vi "Impulse_Correlation.vi"(0 "Head Velocity":dbl[][](array[numeric])=array6400x4[25600 elements] format="%.2f", 2 "Trigger":T1(ring)=enum."Falling Edge", 5 "Cross-Correlation":bool, 7 "Impulse surround":T2={"Pre Impulse (ms)"=150, "Post Impulse (ms) "=150, "Pitch/Roll T for RALP/LARP"=15.0} {"Pitch/Roll T for RALP/LARP" format="%.2f"}, 9 "First Pass Criterea":T5={"Minimum Threshold"=100.0, "Width (ms)"=50, "Maximum Threshold"=100.0} {"Maximum Threshold" format="%.2f"; "Minimum Threshold" format="%.2f"}, 11 "Sample Rate":dbl format="%.2f", 12 "Other Trigger":bool) -> (4 "Impulse Array":T6(array[cluster]) {"Amplitude offset" format="%.2f"})   [LabVIEW 2013, in "impulse functions.lvlib"]
uses:
  impulse functions.lvlib
  <vilib>/Analysis/2dsp.llb/1D Cross Correlation (DBL).vi
  <vilib>/Analysis/NI_AALPro.lvlib
  <vilib>/Analysis/NI_AALBase.lvlib
  <vilib>/Analysis/3filter.llb/Savitzky-Golay Filter (DBL).vi
panel:
  out "extracted head impulse 3":dbl[][](graph)
  out "extracted head impulse 2":dbl[](graph)
  out "extracted head impulse":dbl[][](graph)
  in  "Peaks/Valleys":enum16{"Peaks", "Valleys"}(ring)
  in  "Impulse":T3 {"Amplitude offset" format="%.2f"}
  in  "Impulse Analysis Params":T4={"unfiltered vel?"=FALSE, "remove offset? (T)"=FALSE, "analysis method"=enum."polynomial fit", "pre-impulse position"=50, "post-impulse position"=50, "HIT axis"=enum."Pitch", "pre-impulse pts"=50, "post-impulse pts"=50, "polynomial order"=15, "algorithm"=enum."Givens"}
  # "Copyright Americo A. Migliaccio (c) 2002 All Rights Reserved by Author"
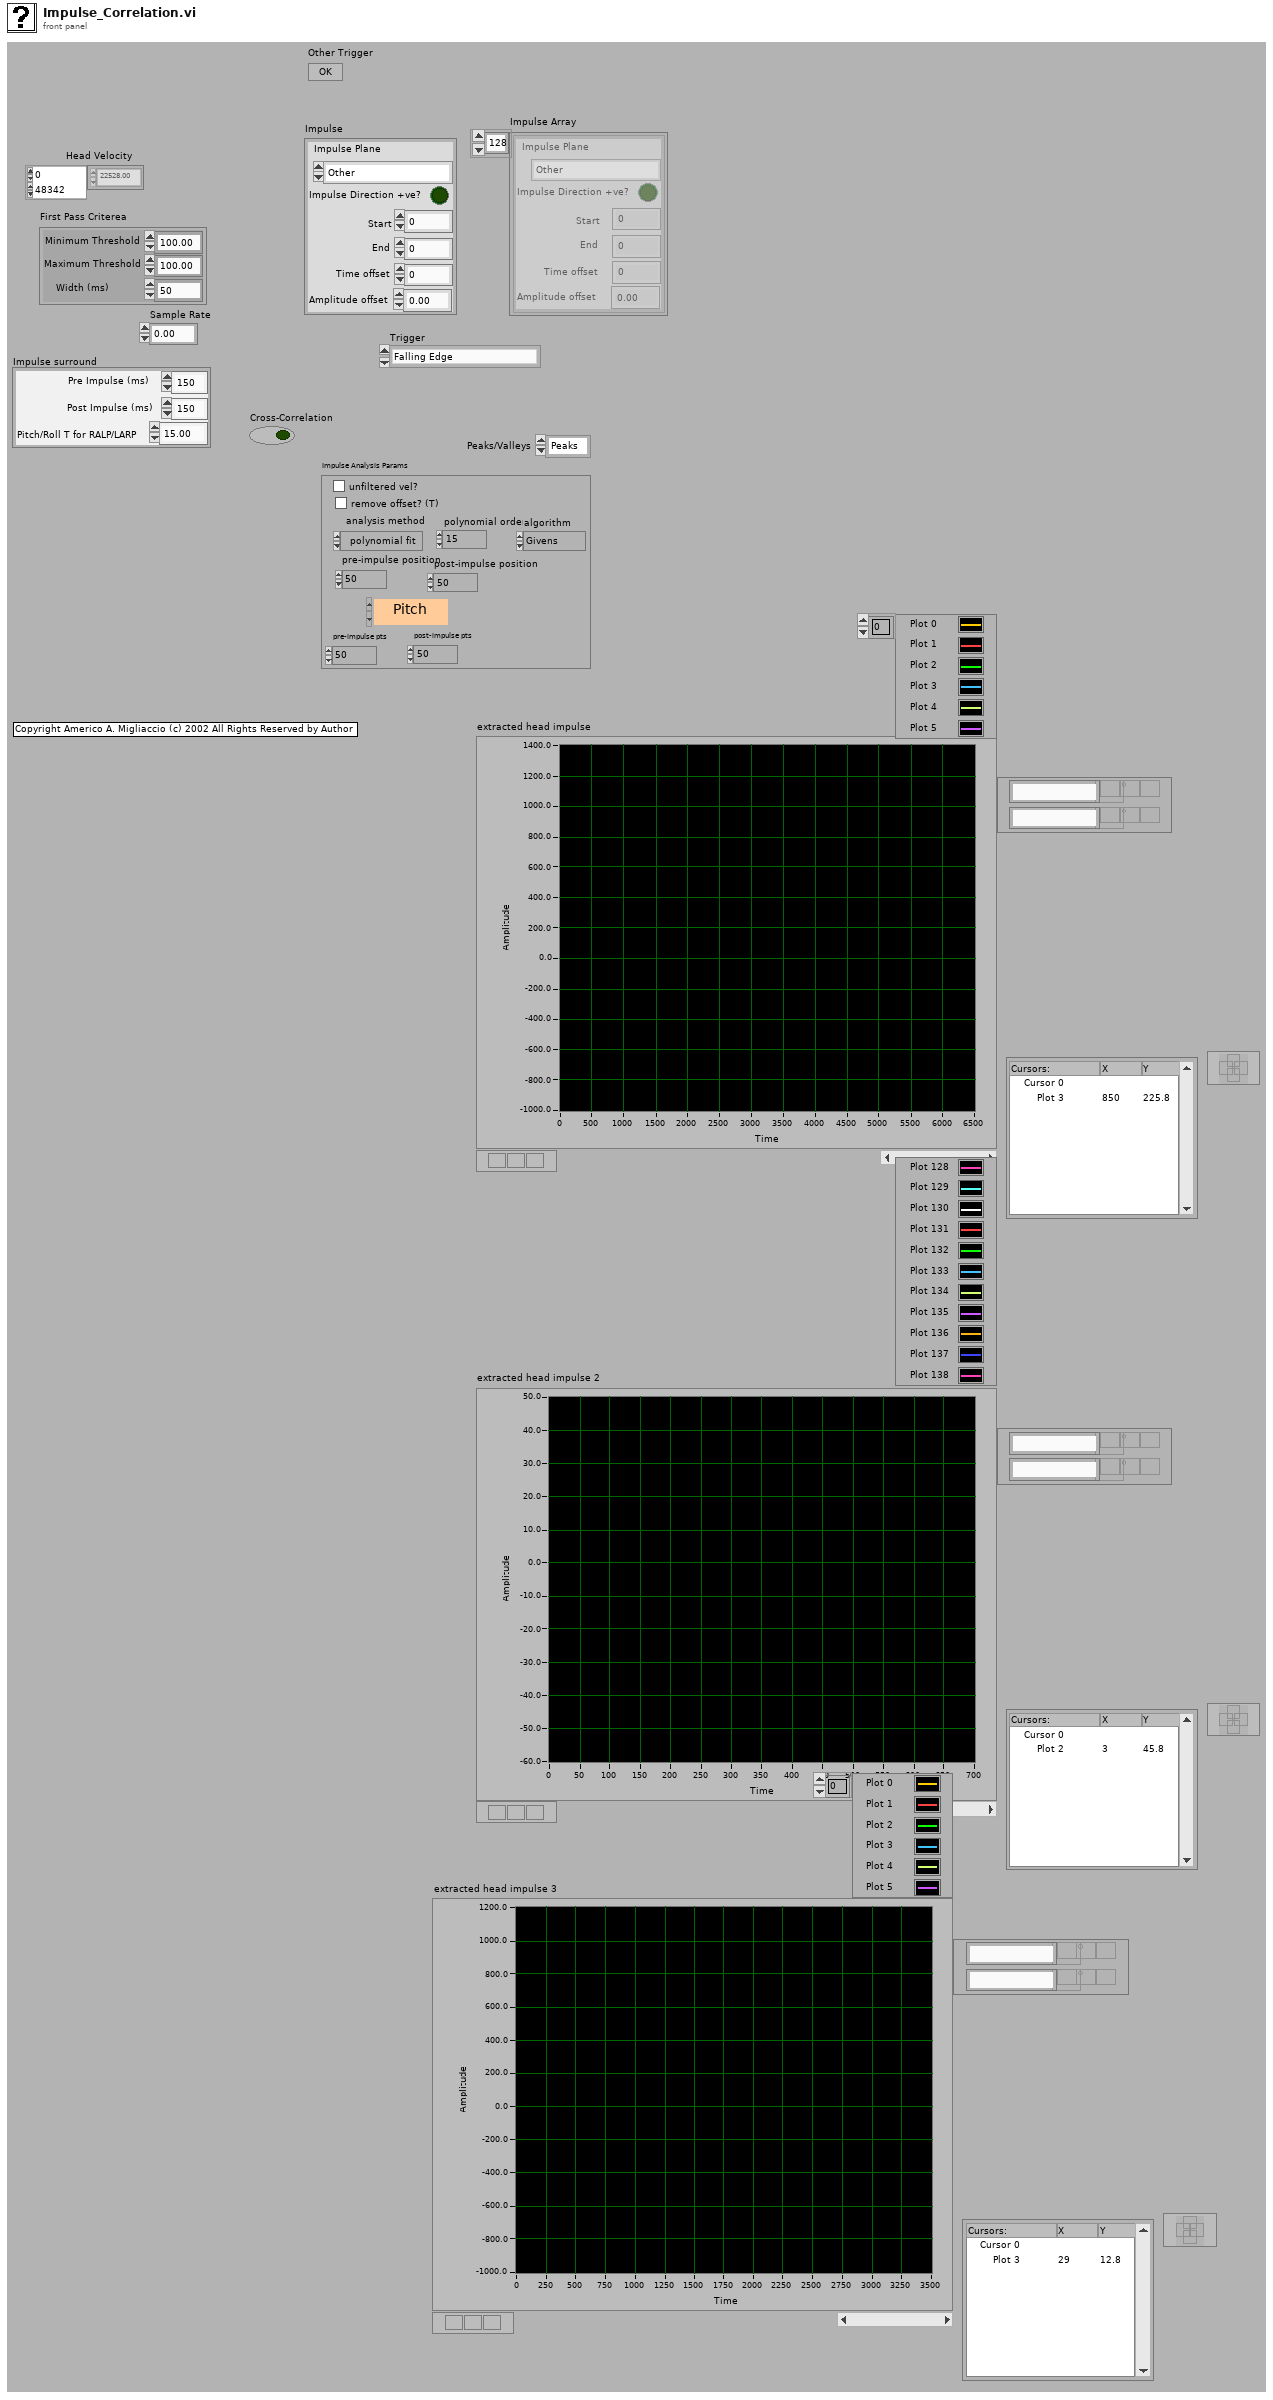
[diagram p1: front panel]
types:
  T1 = enum16{"Peak Detektion", "Rising Edge", "Falling Edge", "Rising Edge (multiple)", "Falling Edge (multiple)"}
  T2 = cluster{"Pre Impulse (ms)":i32, "Post Impulse (ms) ":i32, "Pitch/Roll T for RALP/LARP":dbl}
  T3 = cluster{"Start":i32, "End":i32, "Impulse Plane":enum16{"Other", "Yaw", "Pitch", "Roll", "LARP", "RALP"}, "Impulse Direction +ve?":bool, "Time offset":i32, "Amplitude offset":dbl}
  T4 = cluster{"unfiltered vel?":bool, "remove offset? (T)":bool, "analysis method":enum16{"original", "polynomial fit"}, "pre-impulse position":i32, "post-impulse position":i32, "HIT axis":enum16{"Yaw", "Pitch", "Roll"}, "pre-impulse pts":i32, "post-impulse pts":i32, "polynomial order":i32, "algorithm":enum32{"SVD", "Givens", "Givens2", "Householder", "LU Decomposition", "Cholesky"}}
  T5 = cluster{"Minimum Threshold":dbl, "Width (ms)":i32, "Maximum Threshold":dbl}
  T6 = cluster{"Start":i32, "End":i32, "Impulse Plane":enum16{"Other", "Yaw", "Pitch", "Roll", "LARP", "RALP"}, "Impulse Direction +ve?":bool, "Time offset":i32, "Amplitude offset":dbl}[]
  T7 = cluster{"baseline intercept":dbl, "impulse peak X":dbl, "len":i32, "+ve ?":bool, "peak velocity":dbl}
  T8 = enum16{"Other", "Yaw", "Pitch", "Roll", "LARP", "RALP"}
  T9 = cluster{"Impulse Plane":enum16{"Other", "Yaw", "Pitch", "Roll", "LARP", "RALP"}, "Impulse Direction +ve?":bool}
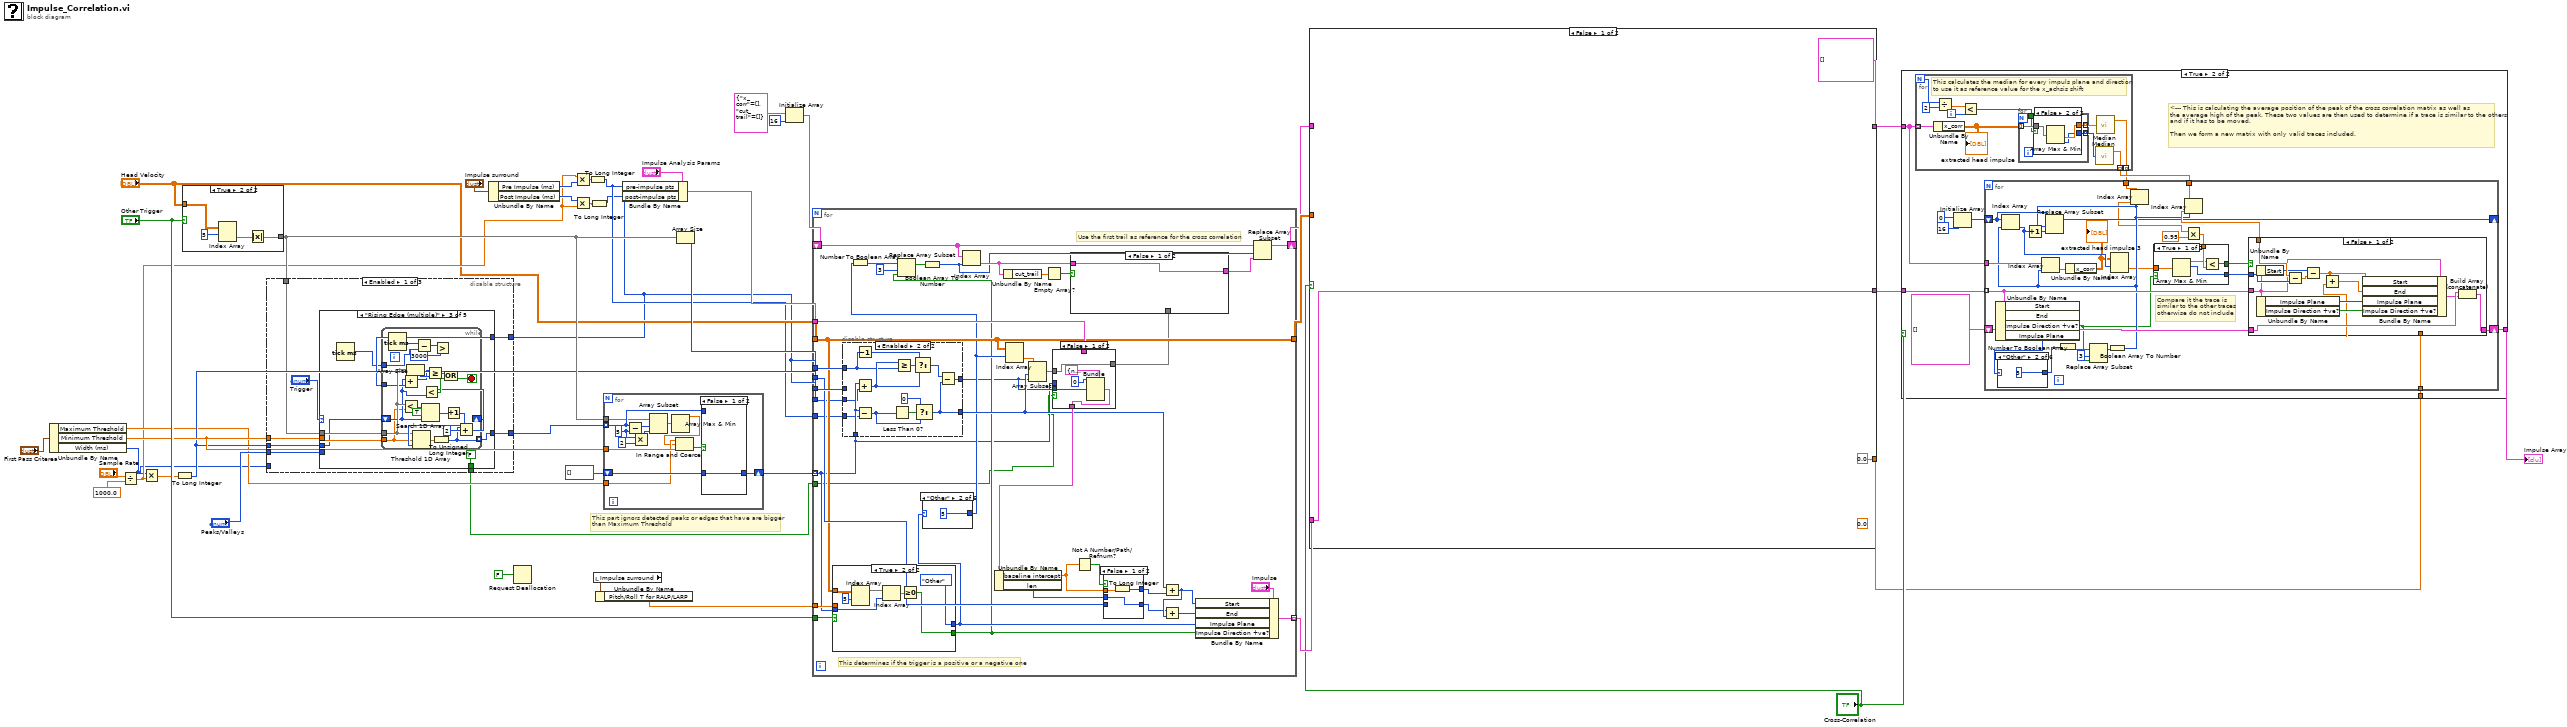
[diagram p0: block diagram]
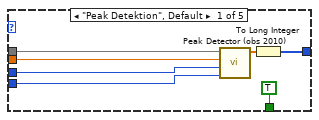
[diagram p2: hidden frame]
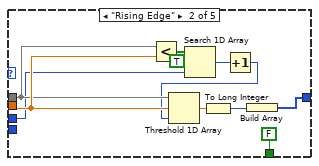
[diagram p3: hidden frame]
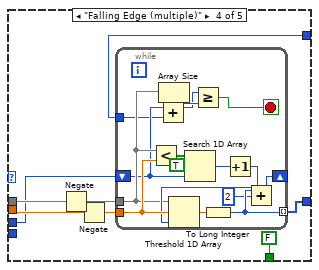
[diagram p4: hidden frame]
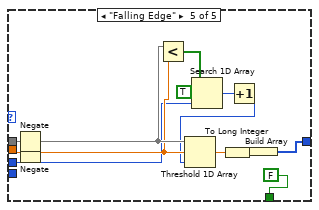
[diagram p5: hidden frame]
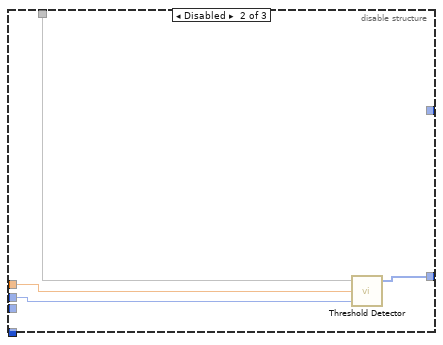
[diagram p6: hidden frame]
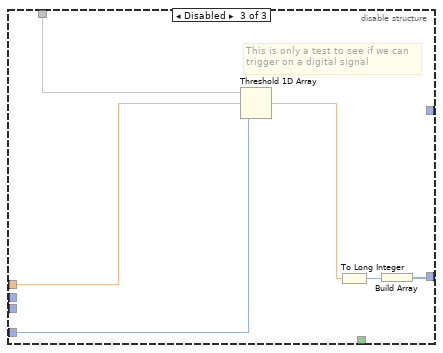
[diagram p7: hidden frame]
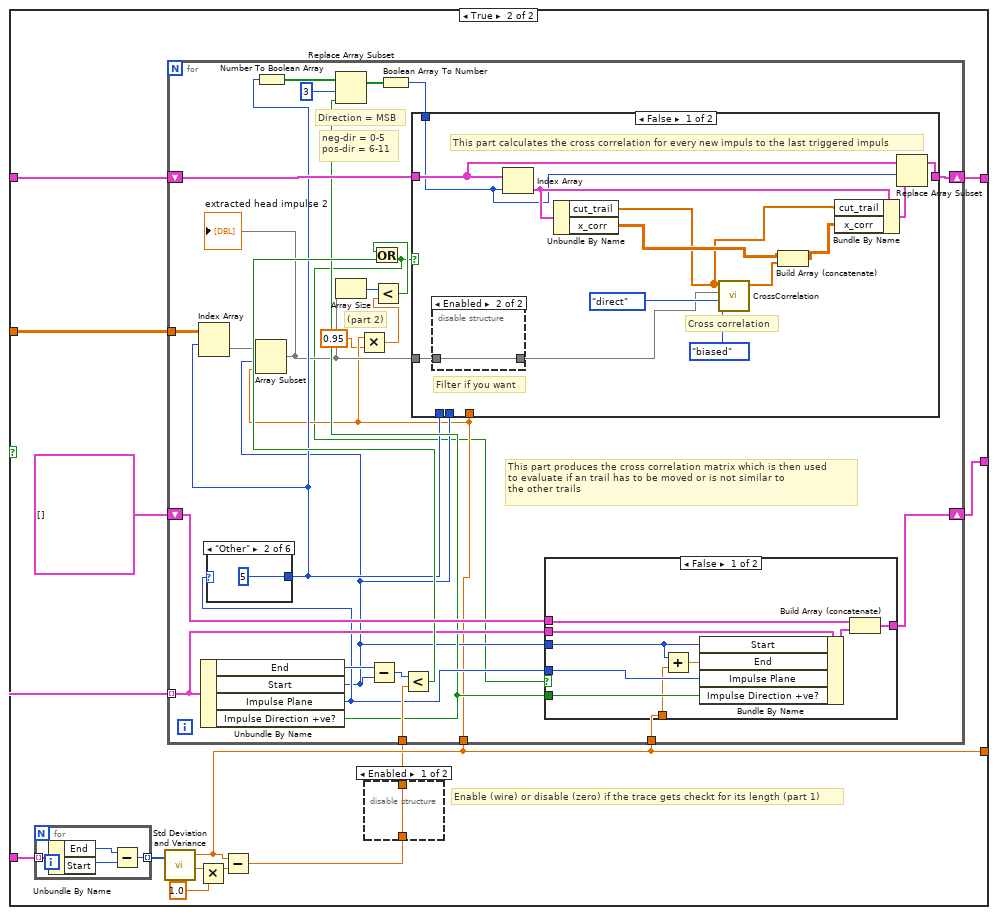
[diagram p8: hidden frame]
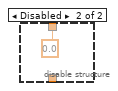
[diagram p9: hidden frame]
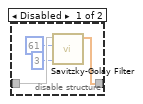
[diagram p10: hidden frame]
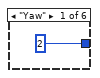
[diagram p12: hidden frame]
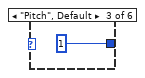
[diagram p13: hidden frame]
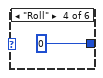
[diagram p14: hidden frame]
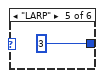
[diagram p15: hidden frame]
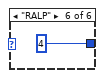
[diagram p16: hidden frame]
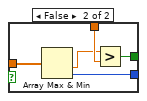
[diagram p19: hidden frame]
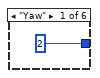
[diagram p20: hidden frame]
diagram:
  # "This part ignors detected peaks or edges that have are bigger \nthan Maximum Threshold"
  n1 = Unbundle By Name("First Pass Criterea") -> ("Maximum Threshold"=w24:dbl, "Minimum Threshold"=w29:dbl, "Width (ms)"=w5:i32)
  n2 = Divide(x="Sample Rate", y=1000.0 ("x")) -> (x/y=w19:dbl)
  n3 = Multiply(x=w5, y=w19) -> (x*y=w18:dbl)
  n4 = To Long Integer(number=w18) -> (32bit integer=w27:i32)
  n5 = case shown="True" "Other Trigger" {
    tunnel: [w46 w47] -> w36
    tunnel: "Head Velocity" -> [w42 w49]
    frame False {
      n6 = Array Subset(array=w42, index (row)=0 ("Array Index"), length (row)=3 ("Array Length")) -> (w43:dbl[][])  [unwired: 2 in]
      n7 = call "norm 3D array.vi"("Vector"=w43) -> ("|x|"=w46:dbl[])  [unwired: 1 in, 1 out]
    }
    frame True {
      n8 = Index Array(array=w49, index (row)=5 ("Array Index")) -> (element=w48:dbl[])  [unwired: 1 in]
      n9 = Absolute Value(x=w48) -> (abs(x)=w47:dbl[])
    }
  }
  n10 = Unbundle By Name("Impulse surround") -> ("Pre Impulse (ms)"=w21:i32, "Post Impulse (ms)"=w20:i32)
  n11 = Request Deallocation(FALSE ("flag")) -> ()
  n12 = Multiply(x=w19, y=w21) -> (x*y=w22:dbl)
  n13 = Multiply(x=w20, y=w19) -> (x*y=w23:dbl)
  n14 = To Long Integer(number=w22) -> (32bit integer=w3:i32)
  n15 = To Long Integer(number=w23) -> (32bit integer=w1:i32)
  n16 = disable-structure shown="Enabled" {
    disable-tunnel: [w58 w141 w148] -> w41
    disable-tunnel: w36 -> [w57 w144 w150]
    disable-tunnel: w29 -> [w56 w143 w149]
    disable-tunnel: "Peaks/Valleys" -> [w55 _ _]
    disable-tunnel: w27 -> [w54 w142 _]
    disable-tunnel: w5 -> [_ _ w145]
    disable-tunnel: [w52 _ _] -> w2
    disable-tunnel: w1 -> [w51 _ _]
    frame Enabled {
      n17 = case shown="\"Rising Edge (multiple)\"" "Trigger" {
        tunnel: [w64 w74 w83 w112 w137] -> w58
        tunnel: w57 -> [w63 w69 w80 w109 w133]
        tunnel: w56 -> [w62 w72 w81 w110 w138]
        tunnel: w55 -> [w61 _ _ _ _]
        tunnel: w54 -> [w60 w68 w79 w108 w130]
        tunnel: [TRUE FALSE FALSE FALSE FALSE] -> w52
        tunnel: w51 -> [_ _ w78 w105 _]
        frame "Peak Detektion", Default {
          n18 = call <vilib>:"Peak Detector (obs 2010).vi"("peaks/valleys"=w61, "width"=w60, "threshold"=w62, "X"=w63) -> ("Locations"=w65:dbl[])  [unwired: 3 in, 4 out]
          n19 = To Long Integer(number=w65) -> (32bit integer=w64:i32[])
        }
        frame "Rising Edge" {
          n20 = Less?(x=w69, y=w72) -> (x < y?=w71:bool[])
          n21 = Search 1D Array(1D array=w71, element=TRUE, start index (0)=w68) -> (index of element=w67:i32)
          n22 = Increment(x=w67) -> (x+1=w66:i32)
          n23 = Threshold 1D Array(1:w66, 2:w72, 3:w69) -> (0:w76:dbl)
          n24 = To Long Integer(number=w76) -> (32bit integer=w75:i32)
          n25 = Build Array(w75) -> (w74:i32[])
        }
        frame "Rising Edge (multiple)" {
          n26 = Tick Count (ms)() -> (millisecond timer value=w77:u32)
          n27 = while {
            tunnel: [w85] -> w83 mode=indexing
            tunnel: w81 -> [w86]
            tunnel: w80 -> [w99]
            shift-right: [w84] -> _
            shift-left: w79 -> [w94]
            tunnel: w78 -> [w95]
            tunnel: w77 -> [w91]
            stop <- w87 stop-if-true
            n28 = Tick Count (ms)() -> (millisecond timer value=w90:u32)
            n29 = Add(x=w94, y=w95) -> (x+y=w96:u32)
            n30 = Less?(x=w99, y=w86) -> (x < y?=w103:bool[])
            n31 = Array Size(array=w99) -> (size(s)=w98:i32)
            n32 = Subtract(x=w90, y=w91) -> (x-y=w89:u32)
            n33 = Search 1D Array(1D array=w103, element=TRUE, start index (0)=w94) -> (index of element=w101:i32)
            n34 = Greater Or Equal?(x=w96, y=w98) -> (x >= y?=w93:bool)
            n35 = Greater?(x=w89, y=u32 3000) -> ()  [unwired: 1 out]
            n36 = Increment(x=w101) -> (x+1=w100:i32)
            n37 = Threshold 1D Array(1:w100, 2:w86, 3:w99) -> (0:w104:dbl)
            n38 = To Unsigned Long Integer(number=w104) -> (unsigned 32bit integer=w85:u32)
            n39 = Add(x=w85, y=2) -> (x+y=w84:u32)
            n40 = Less?(x=w84, y=w94) -> (x < y?=w92:bool)
            n41 = Compound Arithmetic op=OR(w93, w92) -> (w87:bool)
          }
        }
        frame "Falling Edge (multiple)" {
          n42 = Negate(x=w109) -> (-x=w107:dbl[])
          n43 = Negate(x=w110) -> (-x=w106:dbl)
          n44 = while {
            tunnel: [w117] -> w112 mode=indexing
            tunnel: w106 -> [w126]
            tunnel: w107 -> [w121]
            shift-right: [w118] -> _
            shift-left: w108 -> [w119]
            tunnel: w105 -> [w113]
            stop <- w115 stop-if-true
            n45 = Less?(x=w121, y=w126) -> (x < y?=w125:bool[])
            n46 = Add(x=w119, y=w113) -> (x+y=w114:i32)
            n47 = Array Size(array=w121) -> (size(s)=w120:i32)
            n48 = Search 1D Array(1D array=w125, element=TRUE, start index (0)=w119) -> (index of element=w123:i32)
            n49 = Greater Or Equal?(x=w114, y=w120) -> (x >= y?=w115:bool)
            n50 = Increment(x=w123) -> (x+1=w122:i32)
            n51 = Threshold 1D Array(1:w122, 2:w126, 3:w121) -> (0:w127:dbl)
            n52 = To Long Integer(number=w127) -> (32bit integer=w117:i32)
            n53 = Add(x=w117, y=2) -> (x+y=w118:i32)
          }
        }
        frame "Falling Edge" {
          n54 = Negate(x=w133) -> (-x=w132:dbl[])
          n55 = Negate(x=w138) -> (-x=w131:dbl)
          n56 = Less?(x=w132, y=w131) -> (x < y?=w135:bool[])
          n57 = Search 1D Array(1D array=w135, element=TRUE, start index (0)=w130) -> (index of element=w129:i32)
          n58 = Increment(x=w129) -> (x+1=w128:i32)
          n59 = Threshold 1D Array(1:w128, 2:w131, 3:w132) -> (0:w140:dbl)
          n60 = To Long Integer(number=w140) -> (32bit integer=w139:i32)
          n61 = Build Array(w139) -> (w137:i32[])
        }
      }
    }
    frame Disabled {
      n62 = call <vilib>:"Threshold Detector.vi"("width"=w142, "threshold"=w143, "X"=w144) -> ("Indices"=w141:i32[])  [unwired: 2 out]
    }
    frame Disabled {
      # "This is only a test to see if we can\ntrigger on a digital signal"
      n63 = Threshold 1D Array(1:w145, 2:w149, 3:w150) -> (0:w147:dbl)
      n64 = To Long Integer(number=w147) -> (32bit integer=w146:i32)
      n65 = Build Array(w146) -> (w148:i32[])
    }
  }
  n66 = local read "Impulse surround"() -> (w31:T2)
  n67 = Unbundle By Name(w31) -> ("Pitch/Roll T for RALP/LARP"=w30:dbl)
  n68 = for {
    tunnel: w36 -> [w157]
    tunnel: w41 -> [w161] mode=indexing
    shift-right: [w162] -> w39
    shift-left: i32[] [] -> [w163]
    tunnel: w29 -> [w159]
    tunnel: w24 -> [w158]
    w153 = 5 ("y")
    n69 = Subtract(x=w161, y=w153) -> (x-y=w156:u32)
    n70 = Multiply(x=w153, y=2) -> (x*y=w151:i32)
    n71 = Array Subset(array=w157, index=w156, length=w151) -> (w155:dbl[])
    n72 = Array Max & Min(array=w155) -> (max value=w154:dbl)  [unwired: 3 out]
    n73 = In Range and Coerce(upper limit=w158, x=w154, lower limit=w159) -> (In Range?=w160:bool)  [unwired: 1 out]
    n74 = case shown="False" w160 {
      tunnel: w161 -> [_ w166]
      tunnel: w163 -> [w164 w167]
      tunnel: [w164 w165] -> w162
      frame False {
      }
      frame True {
        n75 = Build Array (concatenate)(w167, w166) -> (w165:u32[])
      }
    }
  }
  n76 = Bundle By Name(cluster="Impulse Analysis Params", "pre-impulse pts"=w3, "post-impulse pts"=w1) -> (w33:T4)
  n77 = Array Size(array=w36) -> (size(s)=w38:i32)
  n78 = Initialize Array(cluster{"x_corr":dbl[][], "cut_trail":dbl[]} {"x_corr"=[], "cut_trail"=[]}, 16 ("dimension size")) -> (w7:cluster{"x_corr":dbl[][], "cut_trail":dbl[]}[])
  n79 = for {
    tunnel: w39 -> [w169] mode=indexing
    tunnel: [w194] -> w15 mode=indexing
    tunnel: w27 -> [w205]
    tunnel: w38 -> [w204]
    tunnel: "Head Velocity" -> [w186]
    tunnel: "Other Trigger" -> [w197]
    tunnel: w33 -> [w196]
    tunnel: w30 -> [w193]
    tunnel: w1 -> [w190]
    tunnel: [w186] -> w14
    shift-right: [w185] -> w6
    shift-left: w7 -> [w183]
    tunnel: w3 -> [w172]
    tunnel: w1 -> [w171]
    tunnel: w2 -> [w168]
    # "This determines if the trigger is a positive or a negative one"
    # "Use the first trail as reference for the cross correlation"
    n80 = case shown="True" w197 {
      tunnel: w169 -> [w260 w266]
      tunnel: w186 -> [w259 w265]
      tunnel: [w258 w264] -> w178
      tunnel: [w257 T8."Other" ("Impulse Plane")] -> w187
      tunnel: w193 -> [w256 _]
      frame False {
        n81 = Index Array(array=w259, index (col)=w260) -> (element=w261:dbl[])  [unwired: 1 in]
        n82 = call "Impulse sign and direction 2.vi"("Threshold of either torsion or pitch velocity to determine RALP/LARP"=w256, "Peak X Y Z L R Values"=w261) -> ("Impulse"=w262:T9)  [unwired: 3 in]
        n83 = Unbundle By Name(w262) -> ("Impulse Plane"=w257:T8, "Impulse Direction +ve?"=w258:bool)
      }
      frame True {
        n84 = Index Array(array=w265, index (row)=5 ("Index (row)")) -> (element=w268:dbl[])  [unwired: 1 in]
        n85 = Index Array(array=w268, index=w266) -> (element=w267:dbl)
        n86 = Greater Or Equal To 0?(x=w267) -> (x >= 0?=w264:bool)
      }
    }
    n87 = disable-structure shown="Enabled" {
      disable-tunnel: [w221 w234] -> w170
      disable-tunnel: w205 -> [w219 _]
      disable-tunnel: w204 -> [w218 w232]
      disable-tunnel: [w217 w231] -> w203
      disable-tunnel: w169 -> [w216 w230]
      disable-tunnel: w172 -> [_ w229]
      disable-tunnel: w171 -> [_ w228]
      frame Disabled {
        n88 = Decrement(x=w218) -> (x-1=w225:i32)
        n89 = Add(x=w216, y=w219) -> (x+y=w223:u32)
        n90 = Subtract(x=w216, y=w219) -> (x-y=w220:u32)
        n91 = Less Than 0?(x=w220) -> (x < 0?=w226:bool)
        n92 = Greater Or Equal?(x=w223, y=w218) -> (x >= y?=w227:bool)
        n93 = Select(t=w225, s=w227, f=w223) -> (s? t:f=w222:u32)
        n94 = Select(t=0, s=w226, f=w220) -> (s? t:f=w217:u32)
        n95 = Subtract(x=w222, y=w217) -> (x-y=w221:u32)
      }
      frame Enabled {
        n96 = Decrement(x=w232) -> (x-1=w238:i32)
        n97 = Add(x=w230, y=w228) -> (x+y=w236:u32)
        n98 = Subtract(x=w230, y=w229) -> (x-y=w233:u32)
        n99 = Less Than 0?(x=w233) -> (x < 0?=w239:bool)
        n100 = Greater Or Equal?(x=w236, y=w232) -> (x >= y?=w240:bool)
        n101 = Select(t=w238, s=w240, f=w236) -> (s? t:f=w235:u32)
        n102 = Select(t=0, s=w239, f=w233) -> (s? t:f=w231:u32)
        n103 = Subtract(x=w235, y=w231) -> (x-y=w234:u32)
      }
    }
    n104 = case shown="\"Other\"" w187 {
      tunnel: [2 5 1 0 3 4] -> w179
      frame "Yaw" {
      }
      frame "Other" {
      }
      frame "Pitch", Default {
      }
      frame "Roll" {
      }
      frame "LARP" {
      }
      frame "RALP" {
      }
    }
    n105 = Number To Boolean Array(number=w179) -> (Boolean array=w182:bool[])
    n106 = Replace Array Subset(array=w182, new element=w178, index=3) -> (w180:bool[])
    n107 = Boolean Array To Number(Boolean array=w180) -> (number=w173:i8)
    n108 = Index Array(array=w183, index=w173) -> (element=w176:cluster{"x_corr":dbl[][], "cut_trail":dbl[]})
    n109 = Unbundle By Name(w176) -> ("cut_trail"=w175:dbl[])
    n110 = Index Array(array=w186, index (row)=w179) -> (element=w199:dbl[])  [unwired: 1 in]
    n111 = Array Subset(array=w199, index=w203, length=w170) -> (w198:dbl[])
    n112 = Empty Array?(array=w175) -> (empty?=w177:bool)
    n113 = case shown="False" w168 {
      tunnel: [w208 w215] -> w206
      tunnel: w198 -> [w211 w214]
      tunnel: w196 -> [_ w213]
      tunnel: [w211 w212] -> w174
      tunnel: w170 -> [w209 _]
      tunnel: w169 -> [_ _]
      frame False {
        n114 = Bundle(cluster=T7 {"baseline intercept"=nan, "impulse peak X"=0.0, "len"=2147483647, "+ve ?"=TRUE, "peak velocity"=1.0} ("impulse analysis results"), "baseline intercept"=0, "len"=w209) -> (w208:T7)  [unwired: 3 in]
      }
      frame True {
        n115 = call "AnalyseHeadImpulse2.vi"("head velocity"=w214, "Impulse Analysis Params"=w213) -> ("extracted head impulse"=w212:dbl[], "impulse analysis results"=w215:T7)  [unwired: 9 in, 3 out]
      }
    }
    n116 = Unbundle By Name(w206) -> ("baseline intercept"=w191:dbl, "len"=w188:i32)
    n117 = case shown="False" w177 {
      tunnel: [w241 w244] -> w184
      tunnel: w176 -> [w241 w243]
      tunnel: w174 -> [_ w242]
      frame False {
      }
      frame True {
        n118 = Bundle By Name(cluster=w243, "cut_trail"=w242) -> (w244:cluster{"x_corr":dbl[][], "cut_trail":dbl[]})
      }
    }
    n119 = Not A Number/Path/Refnum?(number/path/refnum=w191) -> (NaN/Path/Refnum?=w192:bool)
    n120 = case shown="False" w192 {
      tunnel: [w252 0 ("y")] -> w202
      tunnel: w191 -> [w253 _]
      tunnel: w190 -> [_ w254]
      tunnel: [w251 w254] -> w189
      tunnel: w188 -> [w251 _]
      frame False {
        n121 = To Long Integer(number=w253) -> (32bit integer=w252:i32)
      }
      frame True {
      }
    }
    n122 = Add(x=w203, y=w202) -> (x+y=w200:u32)
    n123 = Add(x=w189, y=w200) -> (x+y=w201:u32)
    n124 = Bundle By Name(cluster="Impulse", "Start"=w200, "End"=w201, "Impulse Plane"=w187, "Impulse Direction +ve?"=w178) -> (w194:T3)
    n125 = Replace Array Subset(array=w183, new element=w184, index=w173) -> (w185:cluster{"x_corr":dbl[][], "cut_trail":dbl[]}[])
  }
  n126 = case shown="False" "Cross-Correlation" {
    tunnel: w15 -> [w272 w283]
    tunnel: w14 -> [_ w281]
    tunnel: [cluster{"x_corr":dbl[][], "cut_trail":dbl[]}[] [] w280] -> w13
    tunnel: [w272 w279] -> w12
    tunnel: [0.0 ("mean") w278] -> w10
    tunnel: w6 -> [_ w273]
    frame False {
      (unwired) 0.0
    }
    frame True {
      # "Enable (wire) or disable (zero) if the trace gets checkt for its length (part 1)"
      n127 = for {
        tunnel: w283 -> [w353] mode=indexing
        tunnel: [w350] -> w284 mode=indexing
        n128 = Unbundle By Name(w353) -> ("End"=w352:i32, "Start"=w351:i32)
        n129 = Subtract(x=w352, y=w351) -> (x-y=w350:i32)
      }
      n130 = call <vilib>:"Std Deviation and Variance.vi"("X"=w284) -> ("mean"=w278:dbl, "standard deviation"=w285:dbl)  [unwired: 1 in, 1 out]
      n131 = Multiply(x=w285, y=1.0) -> (x*y=w277:dbl)
      n132 = Subtract(x=w278, y=w277) -> (x-y=w275:dbl)
      n133 = disable-structure shown="Enabled" {
        disable-tunnel: w275 -> [w286 _]
        disable-tunnel: [w286 0.0] -> w274
        frame Enabled {
        }
        frame Disabled {
        }
      }
      n134 = for {
        shift-right: [w314] -> w280
        shift-left: w273 -> [w313]
        tunnel: w283 -> [w306] mode=indexing
        shift-right: [w308] -> w279
        shift-left: T6 [] -> [w309]
        tunnel: w274 -> [w310]
        tunnel: w281 -> [w298]
        tunnel: w278 -> [w292]
        tunnel: w278 -> [w304]
        # "This part produces the cross correlation matrix which is then used \nto evaluate if an trail has to be moved or is not similar to\nthe other trails"
        # "(part 2)"
        # "neg-dir = 0-5\npos-dir = 6-11"
        # "Direction = MSB"
        n135 = Unbundle By Name(w306) -> ("End"=w312:i32, "Start"=w295:i32, "Impulse Plane"=w305:T8, "Impulse Direction +ve?"=w300:bool)
        n136 = case shown="\"Other\"" w305 {
          tunnel: [2 5 1 0 3 4] -> w297
          frame "Yaw" {
          }
          frame "Other" {
          }
          frame "Pitch", Default {
          }
          frame "Roll" {
          }
          frame "LARP" {
          }
          frame "RALP" {
          }
        }
        n137 = Index Array(array=w298, index (row)=w297) -> (element=w296:dbl[])  [unwired: 1 in]
        n138 = Array Subset(array=w296, index=w295, length=w292) -> (w294:dbl[])
        "extracted head impulse 2" <- w294
        n139 = Number To Boolean Array(number=w297) -> (Boolean array=w303:bool[])
        n140 = Replace Array Subset(array=w303, new element=w300, index=3) -> (w301:bool[])
        n141 = Array Size(array=w294) -> (size(s)=w293:i32)
        n142 = Multiply(x=w292, y=0.95) -> (x*y=w290:dbl)
        n143 = Subtract(x=w312, y=w295) -> (x-y=w311:i32)
        n144 = Less?(x=w293, y=w290) -> (x < y?=w289:bool)
        n145 = Boolean Array To Number(Boolean array=w301) -> (number=w299:i8)
        n146 = Less?(x=w311, y=w310) -> (x < y?=w307:bool)
        n147 = Or(x=w289, y=w307) -> (x .or. y?=w288:bool)
        n148 = case shown="False" w288 {
          tunnel: [w326 w333] -> w314
          tunnel: w313 -> [w325 w333]
          tunnel: w297 -> [_ _]
          tunnel: w295 -> [_ _]
          tunnel: w292 -> [_ _]
          tunnel: w299 -> [w318 _]
          tunnel: w294 -> [w317 _]
          frame False {
            # "Cross correlation"
            # "Filter if you want"
            # "This part calculates the cross correlation for every new impuls to the last triggered impuls"
            n149 = disable-structure shown="Enabled" {
              disable-tunnel: w317 -> [w331 w332]
              disable-tunnel: [w330 w332] -> w316
              frame Disabled {
                n150 = call-poly <vilib>:"Savitzky-Golay Filter.vi"("polynomial order"=3, "side points"=61, "X"=w331) -> ("Filtered X"=w330:dbl[])  [unwired: 7 in, 1 out]
              }
              frame Enabled {
              }
            }
            n151 = Index Array(array=w325, index=w318) -> (element=w322:cluster{"x_corr":dbl[][], "cut_trail":dbl[]})
            n152 = Unbundle By Name(w322) -> ("cut_trail"=w320:dbl[], "x_corr"=w327:dbl[][])
            n153 = call-poly <vilib>:"CrossCorrelation.vi"("normalization"=enum32{"none", "unbiased", "biased"}."biased", "algorithm"=enum32{"direct", "frequency domain"}."direct", "Y"=w316, "X"=w320) -> ("Rxy"=w315:dbl[])  [unwired: 6 in, 1 out]
            n154 = Build Array (concatenate)(w327, w315) -> (w319:dbl[][])
            n155 = Bundle By Name(cluster=w322, "cut_trail"=w320, "x_corr"=w319) -> (w321:cluster{"x_corr":dbl[][], "cut_trail":dbl[]})
            n156 = Replace Array Subset(array=w325, new element=w321, index=w318) -> (w326:cluster{"x_corr":dbl[][], "cut_trail":dbl[]}[])
          }
          frame True {
            # "Do nothing if trace is to short"
          }
        }
        n157 = case shown="False" w288 {
          tunnel: w309 -> [w342 w349]
          tunnel: [w341 w349] -> w308
          tunnel: w306 -> [w348 _]
          tunnel: w300 -> [w347 _]
          tunnel: w305 -> [w346 _]
          tunnel: w295 -> [w344 _]
          tunnel: w304 -> [w343 _]
          frame False {
            n158 = Add(x=w344, y=w343) -> (x+y=w345:dbl)
            n159 = Bundle By Name(cluster=w348, "Start"=w344, "End"=w345, "Impulse Plane"=w346, "Impulse Direction +ve?"=w347) -> (w340:T3)
            n160 = Build Array (concatenate)(w342, w340) -> (w341:T6)
          }
          frame True {
          }
        }
      }
    }
  }
  n161 = case shown="True" "Cross-Correlation" {
    tunnel: w13 -> [_ w363]
    tunnel: w12 -> [w354 w357]
    tunnel: [w354 w356] -> w16
    tunnel: w10 -> [_ w355]
    frame False {
    }
    frame True {
      # "<--- This is calculating the average position of the peak of the cross correlation matrix as well as \nthe average high of the peak. These two values are then used to determine if a trace is similar to the others\nand if it has to be moved. \n\nThen we form a new matrix with only valid traces included."
      n162 = for {
        N -> [w426]
        tunnel: w363 -> [w432] mode=indexing
        tunnel: [w430] -> w364 mode=indexing
        tunnel: [w427] -> w361 mode=indexing
        i -> [w423]
        # "This calculates the median for every impuls plane and direction\nto use it as reference value for the x_achsis shift"
        n163 = Unbundle By Name(w432) -> ("x_corr"=w429:dbl[][])
        "extracted head impulse" <- w429
        n164 = Divide(x=w426, y=2) -> (x/y=w424:dbl)
        n165 = Less?(x=w424, y=w423) -> (x < y?=w422:bool)
        n166 = for {
          tunnel: w429 -> [w436] mode=indexing
          tunnel: [w435] -> w431 mode=indexing
          tunnel: [w434] -> w428 mode=indexing
          tunnel: w422 -> [w433]
          n167 = case shown="False" w433 {
            tunnel: w436 -> [w439 w442]
            tunnel: [w438 w440] -> w435
            tunnel: [w437 w441] -> w434
            frame True {
              n168 = Array Max & Min(array=w439) -> (max value=w437:dbl, max index (indices)=w438:i32)  [unwired: 2 out]
            }
            frame False {
              n169 = Array Max & Min(array=w442) -> (min value=w441:dbl, min index (indices)=w440:i32)  [unwired: 2 out]
            }
          }
        }
        n170 = call <vilib>:"Median.vi"("X"=w431) -> ("median"=w430:dbl)  [unwired: 1 out]
        n171 = call <vilib>:"Median.vi"("X"=w428) -> ("median"=w427:dbl)  [unwired: 1 out]
      }
      n172 = Initialize Array(0, 16 ("dimension size")) -> (w359:i32[])
      n173 = for {
        tunnel: w357 -> [w386] mode=indexing
        tunnel: w364 -> [w381]
        tunnel: w363 -> [w389]
        shift-right: [w385] -> w356
        shift-left: T6 [] -> [w384]
        tunnel: w361 -> [w380]
        shift-right: [w374] -> _
        shift-left: w359 -> [w377]
        tunnel: w355 -> [w373]
        # "Compare it the trace is \nsimilar to the other traces\notherwise do not include"
        n174 = Unbundle By Name(w386) -> ("Impulse Direction +ve?"=w365:bool, "Impulse Plane"=w383:T8)  [unwired: 2 out]
        n175 = case shown="\"Other\"" w383 {
          tunnel: [2 5 1 0 3 4] -> w382
          frame "Yaw" {
          }
          frame "Other" {
          }
          frame "Pitch", Default {
          }
          frame "Roll" {
          }
          frame "LARP" {
          }
          frame "RALP" {
          }
        }
        n176 = Number To Boolean Array(number=w382) -> (Boolean array=w391:bool[])
        n177 = Replace Array Subset(array=w391, new element=w365, index=3) -> (w390:bool[])
        n178 = Boolean Array To Number(Boolean array=w390) -> (number=w376:u32)
        n179 = Index Array(array=w377, index=w376) -> (element=w372:i32)
        n180 = Increment(x=w372) -> (x+1=w375:i32)
        n181 = Index Array(array=w389, index=w376) -> (element=w371:cluster{"x_corr":dbl[][], "cut_trail":dbl[]})
        n182 = Replace Array Subset(array=w377, new element=w375, index=w376) -> (w374:i32[])
        n183 = Unbundle By Name(w371) -> ("x_corr"=w366:dbl[][])
        "extracted head impulse 3" <- w366
        n184 = Index Array(array=w366, index (row)=w372) -> (element=w370:dbl[])  [unwired: 1 in]
        n185 = Index Array(array=w380, index=w376) -> (element=w367:dbl)
        n186 = Index Array(array=w381, index=w376) -> (element=w379:dbl)
        n187 = Multiply(x=w367, y=0.95) -> (x*y=w368:dbl)
        n188 = case shown="True" w365 {
          tunnel: [w396 w401] -> w388
          tunnel: [w395 w397] -> w387
          tunnel: w370 -> [w394 w400]
          tunnel: w368 -> [w393 w399]
          frame True {
            n189 = Array Max & Min(array=w394) -> (max value=w392:dbl, max index (indices)=w395:i32)  [unwired: 2 out]
            n190 = Less?(x=w392, y=w393) -> (x < y?=w396:bool)
          }
          frame False {
            n191 = Array Max & Min(array=w400) -> (min value=w398:dbl, min index (indices)=w397:i32)  [unwired: 2 out]
            n192 = Greater?(x=w398, y=w399) -> (0:w401:bool)
          }
        }
        n193 = case shown="False" w388 {
          tunnel: w387 -> [w419 _]
          tunnel: w379 -> [w420 _]
          tunnel: w386 -> [w412 _]
          tunnel: [w418 w421] -> w385
          tunnel: w384 -> [w417 w421]
          tunnel: w373 -> [w411 _]
          frame False {
            n194 = Unbundle By Name(w412) -> ("Start"=w416:i32)
            n195 = Unbundle By Name(w412) -> ("Impulse Plane"=w414:T8, "Impulse Direction +ve?"=w415:bool)
            n196 = Subtract(x=w420, y=w419) -> (x-y=w410:dbl)
            n197 = Subtract(x=w416, y=w410) -> (x-y=w413:dbl)
            n198 = Add(x=w413, y=w411) -> (x+y=w408:dbl)
            n199 = Bundle By Name(cluster=w412, "Start"=w413, "End"=w408, "Impulse Plane"=w414, "Impulse Direction +ve?"=w415) -> (w409:T3)
            n200 = Build Array (concatenate)(w417, w409) -> (w418:T6)
          }
          frame True {
            # "Impulse seams to defere from the other impulses"
          }
        }
      }
    }
  }
  "Impulse Array" <- w16
